vi "cross_section.vi"(4 "X2":dbl, 6 "X1":dbl, 8 "Y1":dbl, 9 "array":dbl[][](array[numeric]), 11 "Y2":dbl) -> (1 "Array":dbl[](array[numeric]))   [LabVIEW 2013]
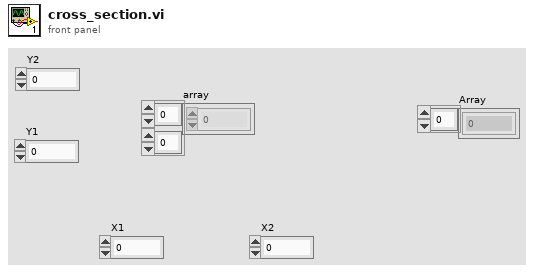
[diagram p1: front panel]
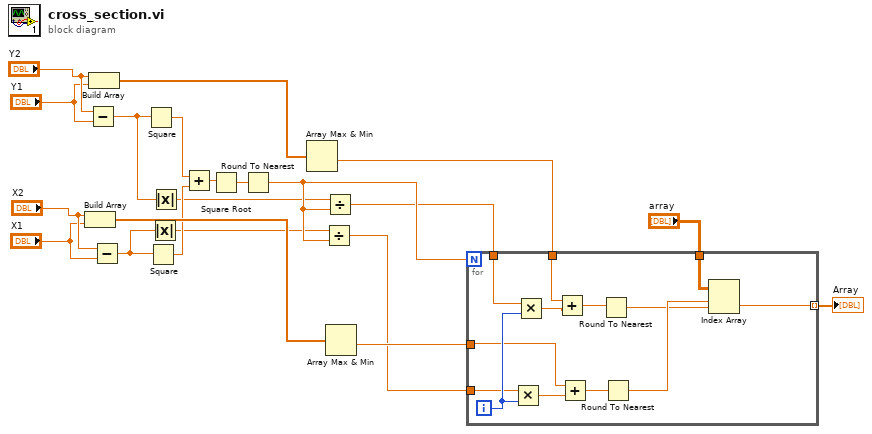
[diagram p0: block diagram]
diagram:
  n1 = Build Array("X2", "X1") -> (w18:dbl[])
  n2 = Subtract(x="Y2", y="Y1") -> (x-y=w2:dbl)
  n3 = Build Array("Y2", "Y1") -> (w10:dbl[])
  n4 = Subtract(x="X2", y="X1") -> (x-y=w4:dbl)
  n5 = Square(x=w2) -> (x^2=w14:dbl)
  n6 = Square(x=w4) -> (x^2=w13:dbl)
  n7 = Absolute Value(x=w4) -> (abs(x)=w3:dbl)
  n8 = Absolute Value(x=w2) -> (abs(x)=w1:dbl)
  n9 = Add(x=w14, y=w13) -> (x+y=w12:dbl)
  n10 = Square Root(x=w12) -> (sqrt(x)=w11:dbl)
  n11 = Round To Nearest(number=w11) -> (nearest integer value=w8:dbl)
  n12 = Array Max & Min(array=w10) -> (min value=w9:dbl)  [unwired: 3 out]
  n13 = Divide(x=w3, y=w8) -> (x/y=w6:dbl)
  n14 = Divide(x=w1, y=w8) -> (x/y=w7:dbl)
  n15 = Array Max & Min(array=w18) -> (min value=w17:dbl)  [unwired: 3 out]
  n16 = for {
    N: w8 -> [_]
    tunnel: "array" -> [w34]
    tunnel: w17 -> [w26]
    tunnel: [w33] -> w5 mode=indexing
    tunnel: w9 -> [w27]
    tunnel: w7 -> [w31]
    tunnel: w6 -> [w30]
    i -> [w32]
    n17 = Multiply(x=w30, y=w32) -> (x*y=w29:dbl)
    n18 = Multiply(x=w31, y=w32) -> (x*y=w28:dbl)
    n19 = Add(x=w27, y=w28) -> (x+y=w25:dbl)
    n20 = Add(x=w26, y=w29) -> (x+y=w24:dbl)
    n21 = Round To Nearest(number=w25) -> (nearest integer value=w22:dbl)
    n22 = Round To Nearest(number=w24) -> (nearest integer value=w23:dbl)
    n23 = Index Array(array=w34, index (row)=w23, index (col)=w22) -> (element=w33:dbl)
  }
  "Array" <- w5
